vi "Initialize.vi"(8 "error in (no error)":errorcluster, 11 "DefaultProjectLoader in":refnum<class "ProjectLoader.lvclass">) -> (0 "error out":errorcluster, 3 "DefaultProjectLoader out":refnum<class "ProjectLoader.lvclass">)   [LabVIEW 2015, in "ProjectLoader.lvclass"]
uses:
  ProjectLoader.lvclass
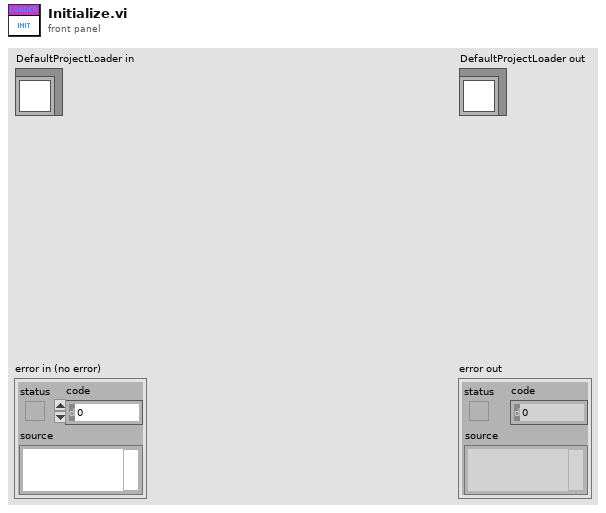
[diagram p1: front panel]
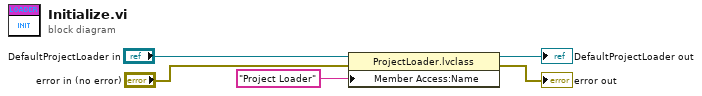
[diagram p0: block diagram]
diagram:
  n1 = property class="ProjectLoader.lvclass"(reference="DefaultProjectLoader in", error in="error in (no error)", "Member Access:Name"="Project Loader" ("Name")) -> (reference out=→"DefaultProjectLoader out":refnum<class "ProjectLoader.lvclass">, error out=→"error out":errorcluster)
